vi "sub_test_FP.vi"() -> ()   [LabVIEW 2018]
panel:
  in  "stop":bool
  out "Numeric":i32
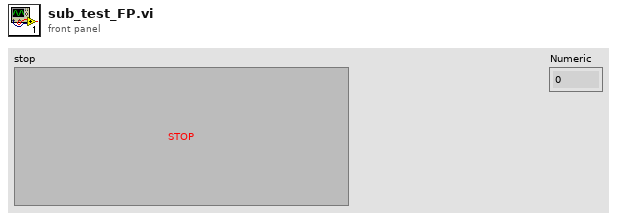
[diagram p1: front panel]
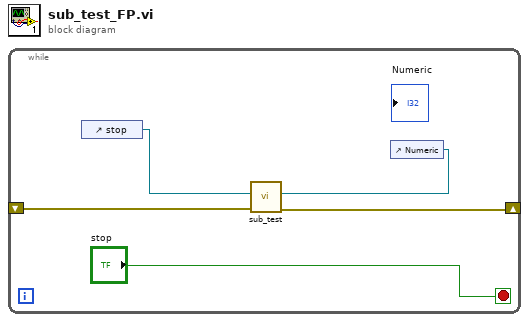
[diagram p0: block diagram]
diagram:
  n1 = while {
    shift-right: [w3] -> _
    shift-left: _ -> [w4]
    stop <- "stop" stop-if-true
    n2 = control-ref of="stop"() -> (w1:refnum<vi>)
    n3 = control-ref of="Numeric"() -> (w5:refnum<vi>)
    n4 = call "sub_test.vi"("Numeric 2"=w5, "error in"=w4, "stop"=w1) -> ("error out"=w3:errorcluster)  [unwired: 8 in]
  }
